vi "Wiimote Calculate Acceleration.vi"(1 "Acceleration 1G Calibration":T1={"Acceleration X"=154.0, "Acceleration Y"=157.0, "Acceleration Z"=152.0}, 2 "Acceleration 0G Calibration":T1={"Acceleration X"=127.0, "Acceleration Y"=131.0, "Acceleration Z"=126.0}, 3 "Acceleration Raw in":T1={"Acceleration X"=112.0, "Acceleration Y"=115.0, "Acceleration Z"=134.0}) -> (0 "Acceleration Calibrated Out":T1={"Acceleration X"=-0.5555555555555556, "Acceleration Y"=-0.6153846153846154, "Acceleration Z"=0.3076923076923077})   [LabVIEW 2011, in "Wiimote.lvlib"]
uses:
  Wiimote.lvlib
  Wiimote Acceleration.ctl
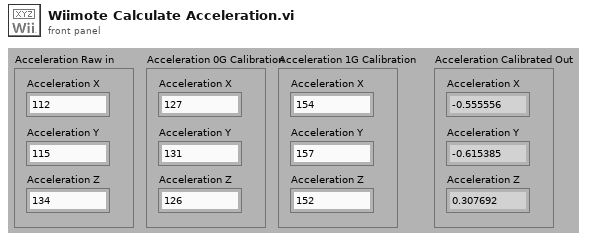
[diagram p1: front panel]
types:
  T1 = typedef "Wiimote.lvlib/Wiimote Acceleration.ctl" = cluster{"Acceleration X":dbl, "Acceleration Y":dbl, "Acceleration Z":dbl}
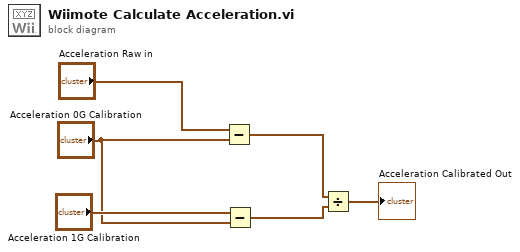
[diagram p0: block diagram]
diagram:
  n1 = Subtract(x="Acceleration Raw in", y="Acceleration 0G Calibration") -> (x-y=w3:T1)
  n2 = Subtract(x="Acceleration 1G Calibration", y="Acceleration 0G Calibration") -> (x-y=w2:T1)
  n3 = Divide(x=w3, y=w2) -> (x/y=→"Acceleration Calibrated Out":T1)
